vi "Agilent DMM Set Trigger Source.vi"(8 "error in (no error)":errorcluster, 10 "Trigger Source":T1, 11 "VISA Resource Name":refnum<visa-resource-name>) -> (0 "error out":errorcluster, 3 "dup VISA Resource Name":refnum<visa-resource-name>)   [LabVIEW 2011]
doc: "This VI for the HP 8753 is used to read the sweep type.\n\n0 LINEAR FREQ\n1 LOG FREQ\n2 LIST FREQ\n3 CW TIME\n4 POWER SWEEP"
uses:
  TypeDefs/Agilent DMM Trigger Source.ctl
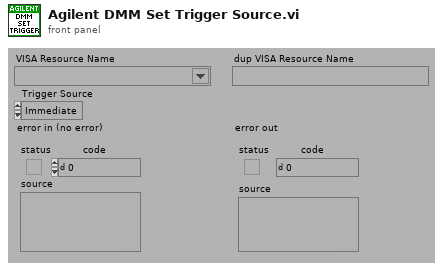
[diagram p1: front panel]
types:
  T1 = typedef "Agilent DMM Trigger Source.ctl" = enum16{"Immediate", "Bus", "External"}
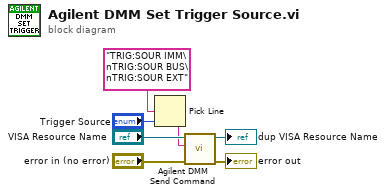
[diagram p0: block diagram]
diagram:
  n1 = Pick Line(multi-line string="TRIG:SOUR IMM\nTRIG:SOUR BUS\nTRIG:SOUR EXT" ("write buffer"), line index="Trigger Source") -> (output string=w1:string)  [unwired: 1 out]
  n2 = call "Agilent DMM Send Command.vi"("error in (no error)"="error in (no error)", "Command"=w1, "VISA Resource Name"="VISA Resource Name") -> ("error out"=→"error out":errorcluster, "dup VISA Resource Name"=→"dup VISA Resource Name":refnum<visa-resource-name>)  [unwired: 2 in, 5 out]
